vi "Save File Four Stations.vi"(0 "File Locations A in":T7, 1 "File Locations B in":T7, 2 "File Locations C in":T7, 3 "File Locations D in":T7, 7 "Error In":errorcluster, 8 "Save Data A":bool, 9 "A Data Array":string[][](array[string]), 10 "Save Data B":bool, 11 "B Data Array":string[][](array[string]), 12 "Save Data C":bool, 13 "C Data Array":string[][](array[string]), 14 "Save Data D":bool, 15 "D Data Array":string[][](array[string]), 17 "Appliance Details":T1[](array[typedef]) {"Dryer"."Dryer Initial IMC Data"."Maximum Weight (lbf)" format="%03_6g"; "Dryer"."Dryer Initial IMC Data"."Average Weight (lbf)" format="%03_6g"; "Dryer"."Dryer Initial IMC Data"."Minimum Weight (lbf)" format="%03_6g"; "Dryer"."Dryer Initial IMC Data"."CEF (lbf/kWh)" format="%03_6g"; "Dryer"."Dryer Initial IMC Data"."Actual Final RMC (%)" format="%03_6g"; "Dryer"."Dryer Initial IMC Data"."Tolerance(%)" format="%0#_6g"; "Dryer"."Dryer Initial IMC Data"."Bone Dry Wt(lbs)" format="%03_6g"; "Dryer"."Dryer Initial IMC Data"."RMC (Desired %)" format="%0#_6g"; "Dryer"."Dryer Initial IMC Data"."Actual Initial RMC (%)" format="%03_6g"; "Dryer"."Dryer Initial IMC Data"."Measured IMC (lbs)" format="%0#_6g"}) -> (18 "Saving A":bool, 20 "File Locations A out":T7, 21 "File Locations B out":T7, 22 "File Locations C out":T7, 23 "File Locations D out":T7, 24 "Saving B":bool, 25 "Saving C":bool, 26 "Saving D":bool, 27 "Error Out":errorcluster)   [LabVIEW 2016]
uses:
  File Setup (Public)/Type Definition/Save File DOE File Path Control.ctl
  File Setup (Public)/Type Definition/Save File DOE Data Save Filepaths.ctl
  File Setup (Public)/Type Definition/Save File DISH Dishwasher Details.ctl
  <vilib>/Platform/fileVersionInfo.llb/FileVersionInformation.ctl
  Washer DOE/Type Definitions/DOE Appliance Common.ctl
  Custom Pallet Controls/Custom Pallet String.ctl
  File Setup (Public)/Type Definition/DPT IMC Data.ctl
  Washer DOE/Type Definitions/DOE Dryer Standard.ctl
  File Setup.lvlib
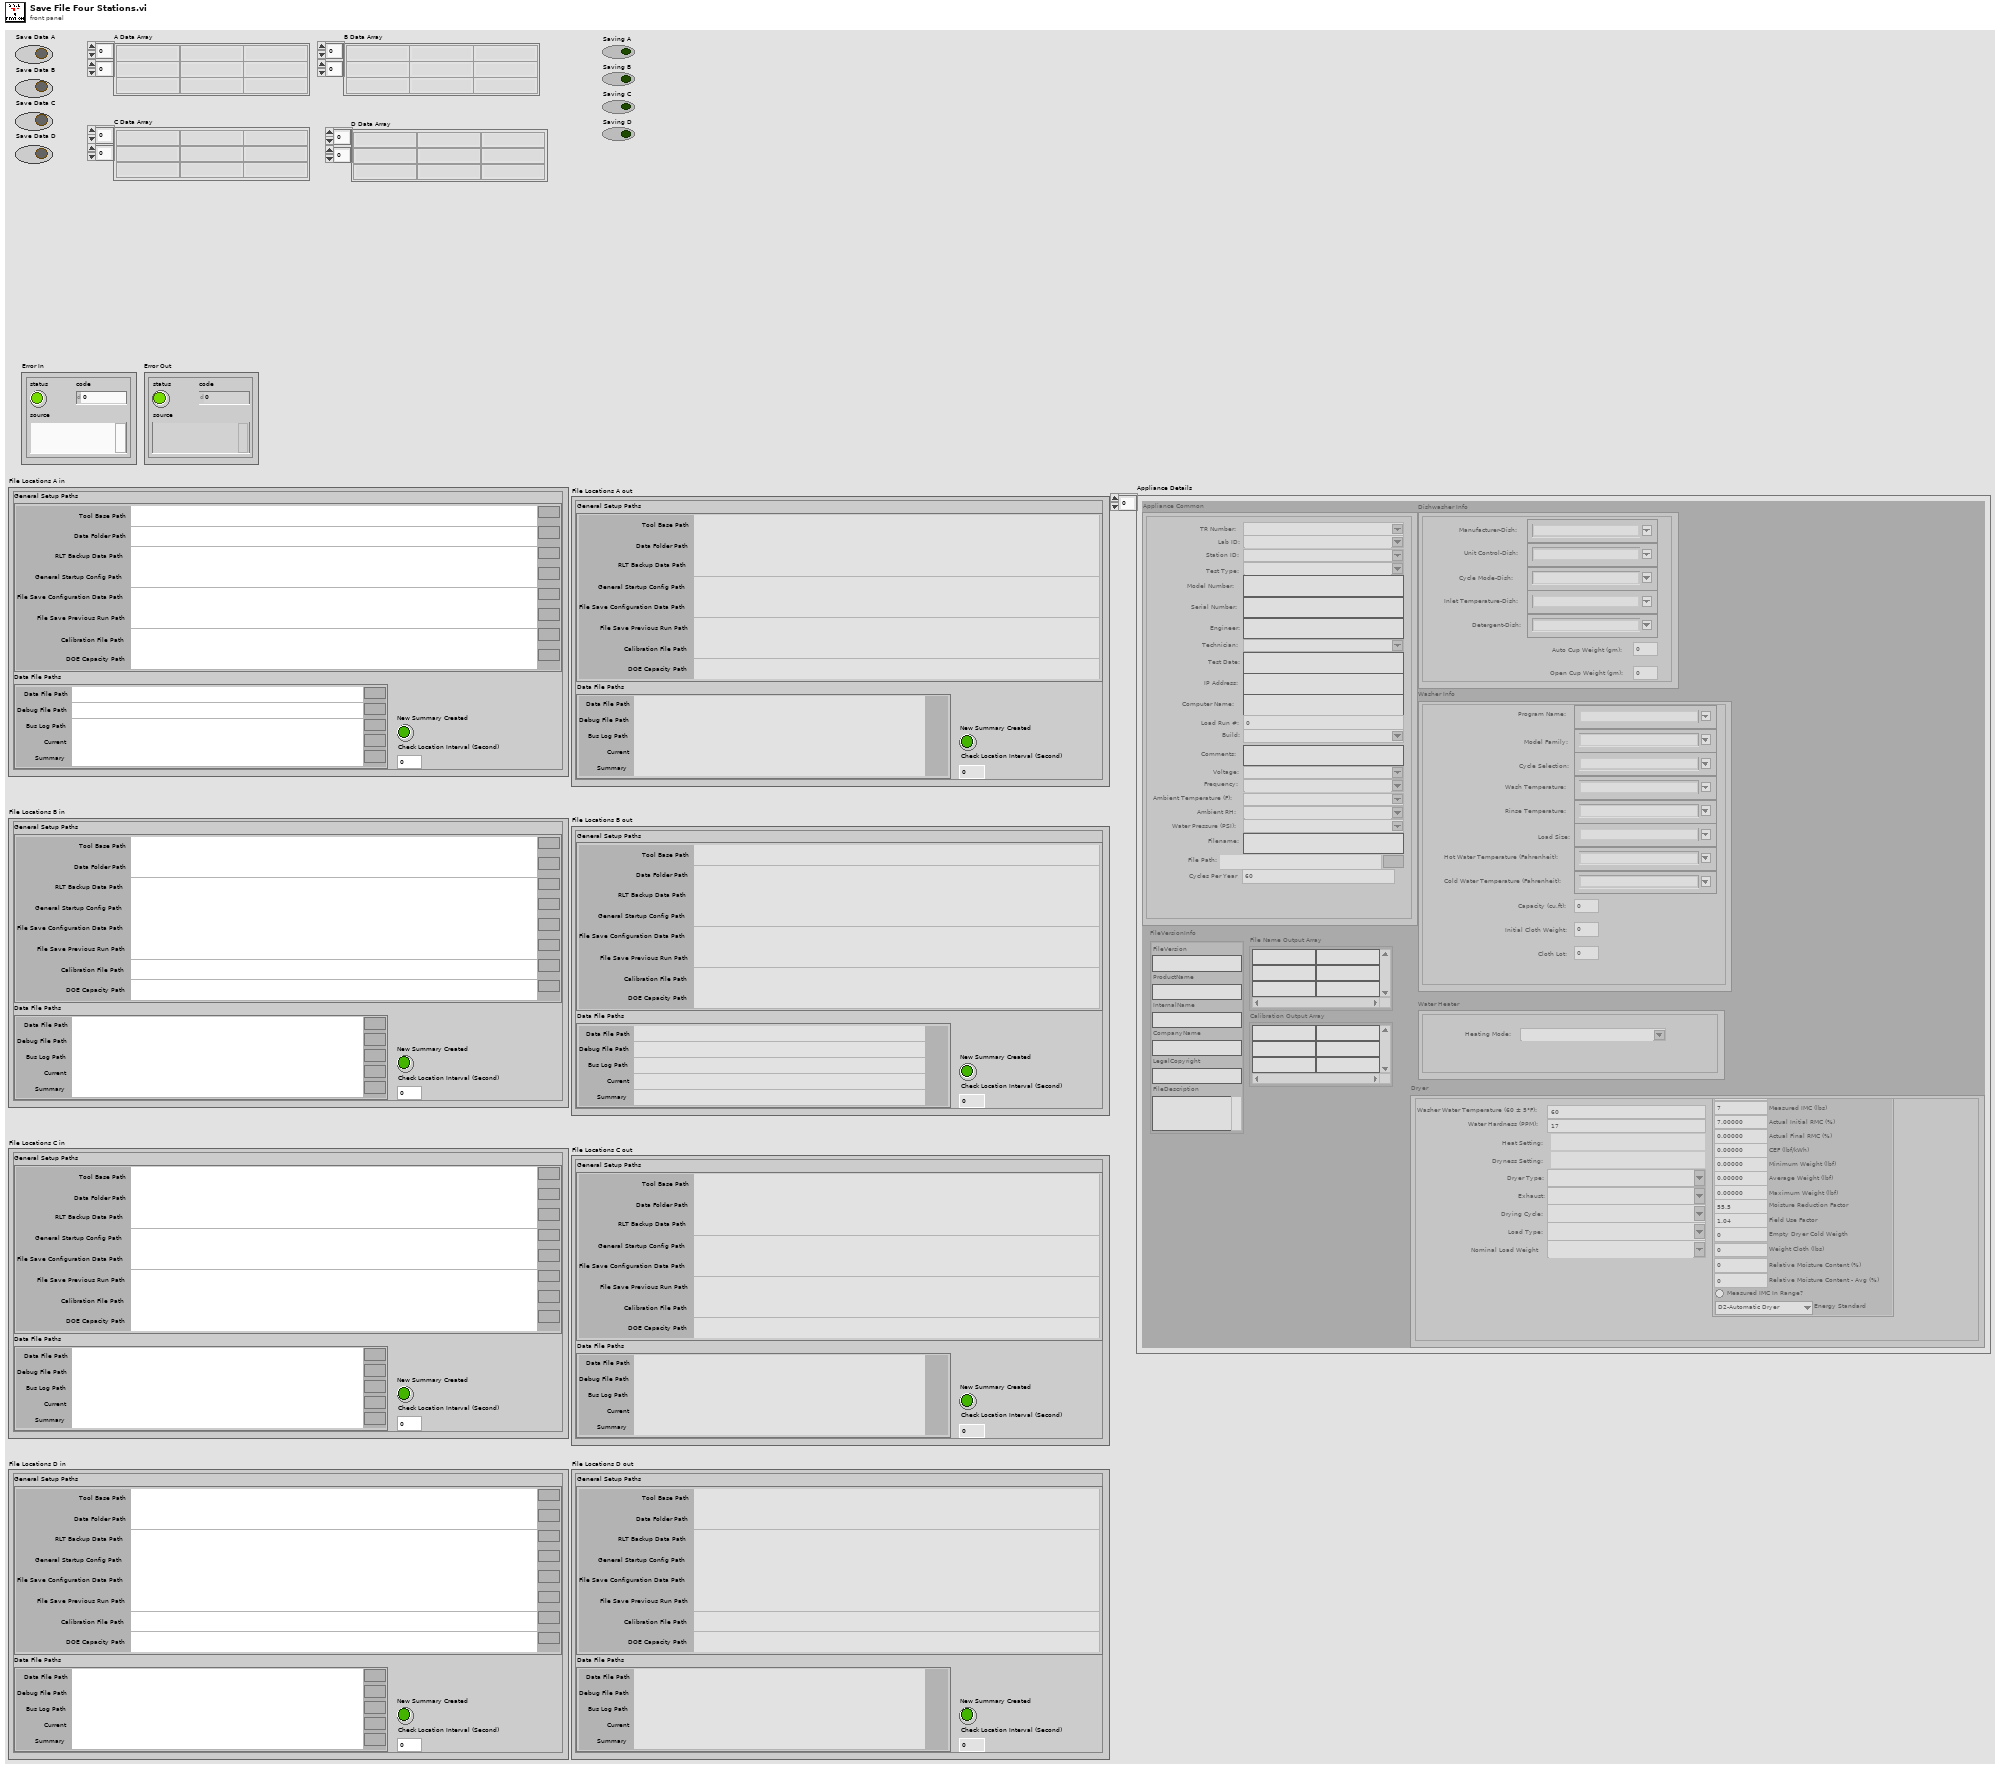
[diagram p1: front panel]
types:
  T1 = typedef "File Setup.lvlib/Save File DISH Dishwasher Details.ctl" = cluster{"FileVersionInfo":T2, "Dishwasher Info":cluster{"Open Cup Weight (gm):":dbl, "Auto Cup Weight (gm):":dbl, "Detergent-Dish:":string, "Inlet Temperature-Dish:":string, "Cycle Mode-Dish:":string, "Unit Control-Dish:":string, "Manufacturer-Dish:":string}, "Washer Info":cluster{"Hot Water Temperature (Fahrenheit):":string, "Cold Water Temperature (Fahrenheit):":string, "Capacity (cu.ft):":dbl, "Initial Cloth Weight:":dbl, "Cloth Lot:":i32, "Model Family:":string, "Program Name:":string, "Cycle Selection:":string, "Wash Temperature:":string, "Rinse Temperature:":string, "Load Size:":string}, "File Name Output Array":string[][], "Calibration Output Array":string[][], "Appliance Common":T3, "Water Heater":cluster{"Heating Mode:":string}, "Dryer":cluster{"Heat Setting:":T4, "Washer Water Temperature (60 ± 5°F):":u16, "Water Hardness (PPM):":u16, "Dryness Setting:":T4, "Dryer Type:":string, "Exhaust:":string, "Drying Cycle:":string, "Load Type:":string, "Nominal Load Weight":string, "Dryer Initial IMC Data":T5}}
  T2 = typedef "FileVersionInformation.ctl" = cluster{"FileVersion":string, "ProductName":string, "InternalName":string, "CompanyName":string, "LegalCopyright":string, "FileDescription":string}
  T3 = typedef "DOE Appliance Common.ctl" = cluster{"Engineer:":string, "Model Number:":string, "Serial Number:":string, "Comments:":string, "Station ID:":string, "Technician:":string, "TR Number:":string, "Lab ID:":string, "Voltage:":string, "Water Pressure (PSI):":string, "Test Date:":string, "Computer Name:":string, "IP Address:":string, "Ambient RH:":string, "Frequency:":string, "Build:":string, "Filename:":string, "Test Type:":string, "Load Run #:":i32, "Ambient Temperature (F):":string, "File Path:":path, "Cycles Per Year":u32}
  T4 = typedef "Custom Pallet String.ctl" = string
  T5 = typedef "DPT IMC Data.ctl" = cluster{"Measured IMC (lbs)":dbl, "Actual Initial RMC (%)":dbl, "RMC (Desired %)":dbl, "Bone Dry Wt(lbs)":dbl, "Tolerance(%)":dbl, "Actual Final RMC (%)":dbl, "CEF (lbf/kWh)":dbl, "Minimum Weight (lbf)":dbl, "Average Weight (lbf)":dbl, "Maximum Weight (lbf)":dbl, "Measured IMC In Range?":bool, "Moisture Reduction Factor":dbl, "Field Use Factor":dbl, "Empty Dryer Cold Weigth":dbl, "Energy Standard":T6, "Weight Cloth (lbs)":dbl, "Relative Moisture Content (%)":dbl, "Relative Moisture Content - Avg (%)":dbl}
  T6 = typedef "DOE Dryer Standard.ctl" = enum16{"D2-Automatic Dryer", "D2-Timer Dryer", "D1-Automatic Dryer", "D1-Timer Dryer", "Other"}
  T7 = typedef "File Setup.lvlib/Save File DOE File Path Control.ctl" = cluster{"General Setup Paths":cluster{"Calibration File Path":path, "DOE Capacity Path":path, "Data Folder Path":path, "RLT Backup Data Path":path, "Tool Base Path":path, "General Startup Config Path":path, "File Save Previous Run Path":path, "File Save Configuration Data Path":path}, "Data File Paths":T8, "New Summary Created":bool, "Check Location Interval (Second)":i32}
  T8 = typedef "File Setup.lvlib/Save File DOE Data Save Filepaths.ctl" = cluster{"Data File Path":path, "Debug File Path":path, "Bus Log Path":path, "Current":path, "Summary":path}
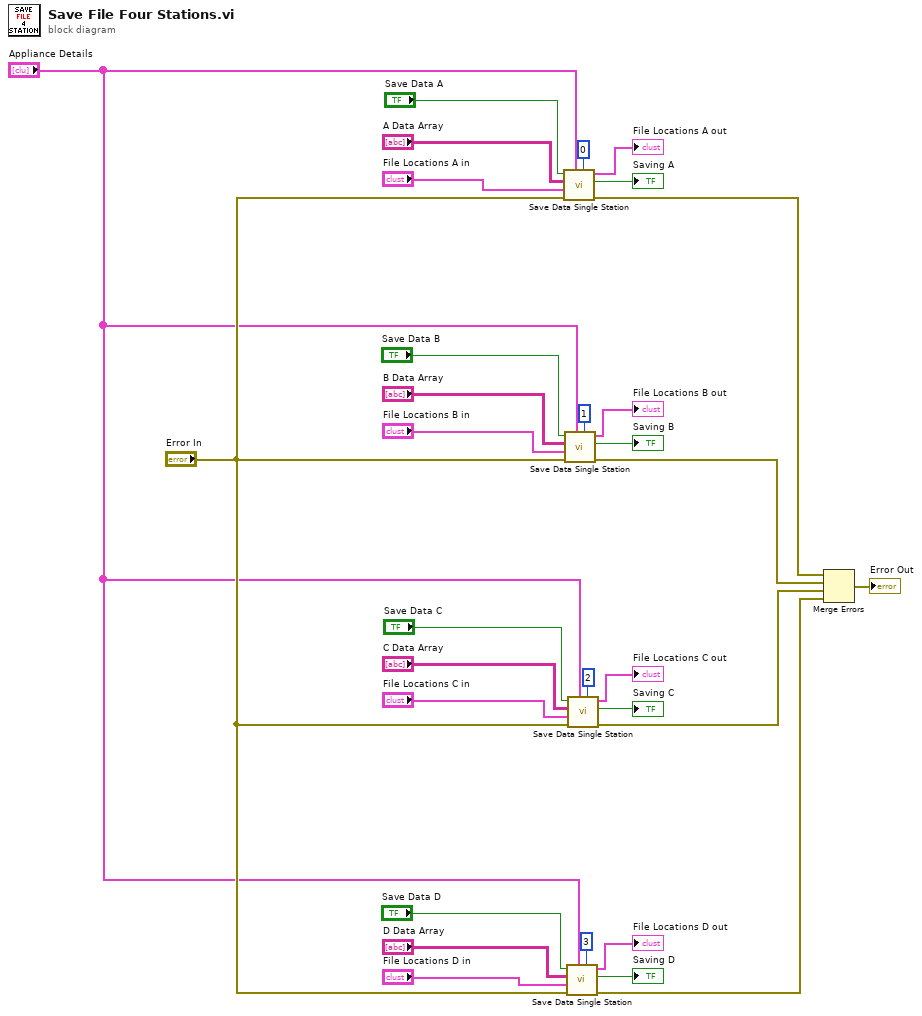
[diagram p0: block diagram]
diagram:
  n1 = call "Save Data Single Station.vi"("index"=0, "Appliance Details"="Appliance Details", "Error In"="Error In", "File Locations in"="File Locations A in", "Data Array"="A Data Array", "Log Data?"="Save Data A") -> ("Error Out"=w10:errorcluster, "Saving"=→"Saving A":bool, "File Locations out"=→"File Locations A out":T7)  [unwired: 3 in]
  n2 = call "Save Data Single Station.vi"("index"=1, "Appliance Details"="Appliance Details", "Error In"="Error In", "File Locations in"="File Locations B in", "Data Array"="B Data Array", "Log Data?"="Save Data B") -> ("Error Out"=w9:errorcluster, "Saving"=→"Saving B":bool, "File Locations out"=→"File Locations B out":T7)  [unwired: 3 in]
  n3 = call "Save Data Single Station.vi"("index"=3, "Appliance Details"="Appliance Details", "Error In"="Error In", "File Locations in"="File Locations D in", "Data Array"="D Data Array", "Log Data?"="Save Data D") -> ("Error Out"=w7:errorcluster, "Saving"=→"Saving D":bool, "File Locations out"=→"File Locations D out":T7)  [unwired: 3 in]
  n4 = call "Save Data Single Station.vi"("index"=2, "Appliance Details"="Appliance Details", "Error In"="Error In", "File Locations in"="File Locations C in", "Data Array"="C Data Array", "Log Data?"="Save Data C") -> ("Error Out"=w8:errorcluster, "Saving"=→"Saving C":bool, "File Locations out"=→"File Locations C out":T7)  [unwired: 3 in]
  n5 = Merge Errors(w10, w9, w8, w7) -> (→"Error Out":errorcluster)
